vi "updateRobotExtraInfo.vi"(8 "error in (no error)":errorcluster, 9 "ReplayArray":bool[](array[boolean]), 11 "Game in":refnum<class "Game.lvclass">) -> (0 "error out":errorcluster, 1 "delay":dbl, 3 "Game out":refnum<class "Game.lvclass">)   [LabVIEW 2020, in "Game.lvclass"]
uses:
  Game.lvclass
  Robot_class/Robot.lvclass
  Game.lvclass/Game.ctl
  Team_class/Team.lvclass/Team.ctl
  Read AllyRef.vi
  Team_class/Read RobotRef.vi
  Read EnemyRef.vi
  Team_class/Write RobotRef.vi
  Write AllyRef.vi
  Write EnemyRef.vi
  Enemy_class/Enemy.lvclass
  Ally_class/Ally.lvclass
  Utilities_class/Utilities.lvclass
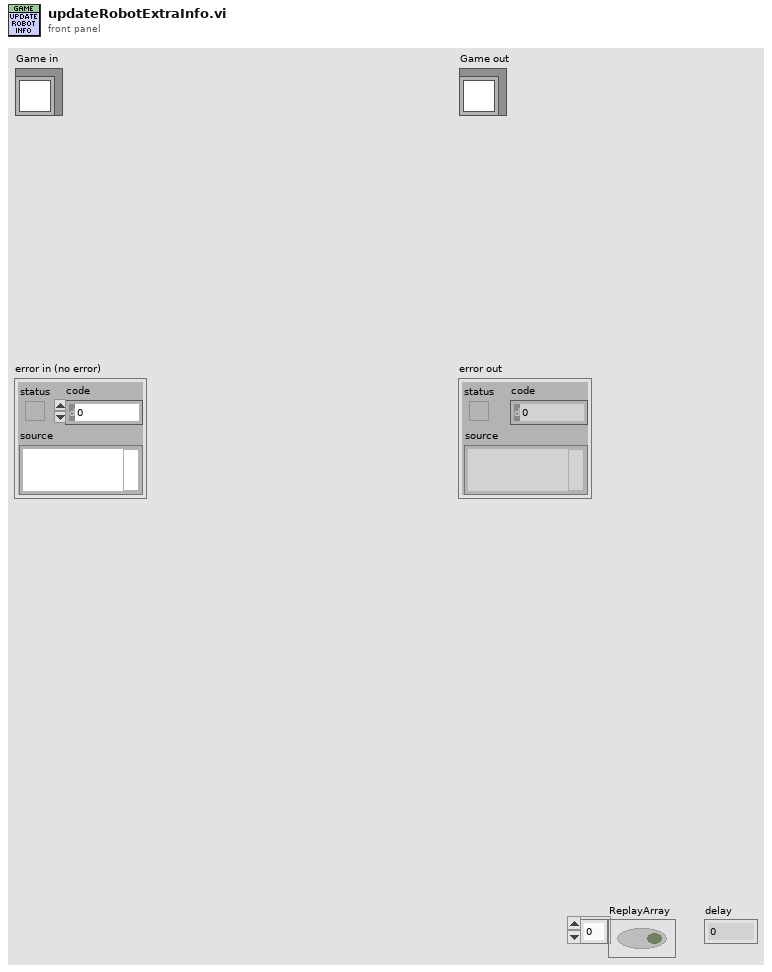
[diagram p1: front panel]
types:
  T1 = typedef "ReplayInfo.ctl" = cluster{"ByteArrayFromVision":u8[], "TimeStampSampledInReplay":string, "ByteArrayFromReferee":u8[], "AllyRobotExtraInfoArray":T2[], "EnemyRobotExtraInfoArray":T2[]}
  T2 = typedef "RobotExtraInfo.ctl" = cluster{"est_vx":dbl, "est_vy":dbl, "id":dbl}
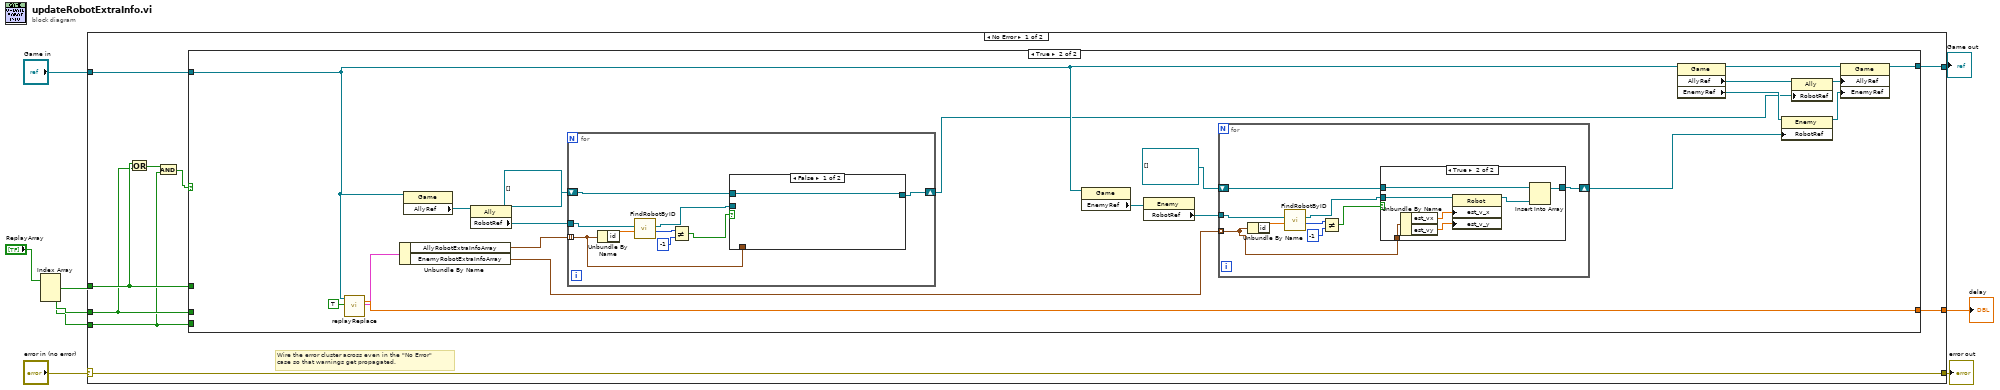
[diagram p0: block diagram]
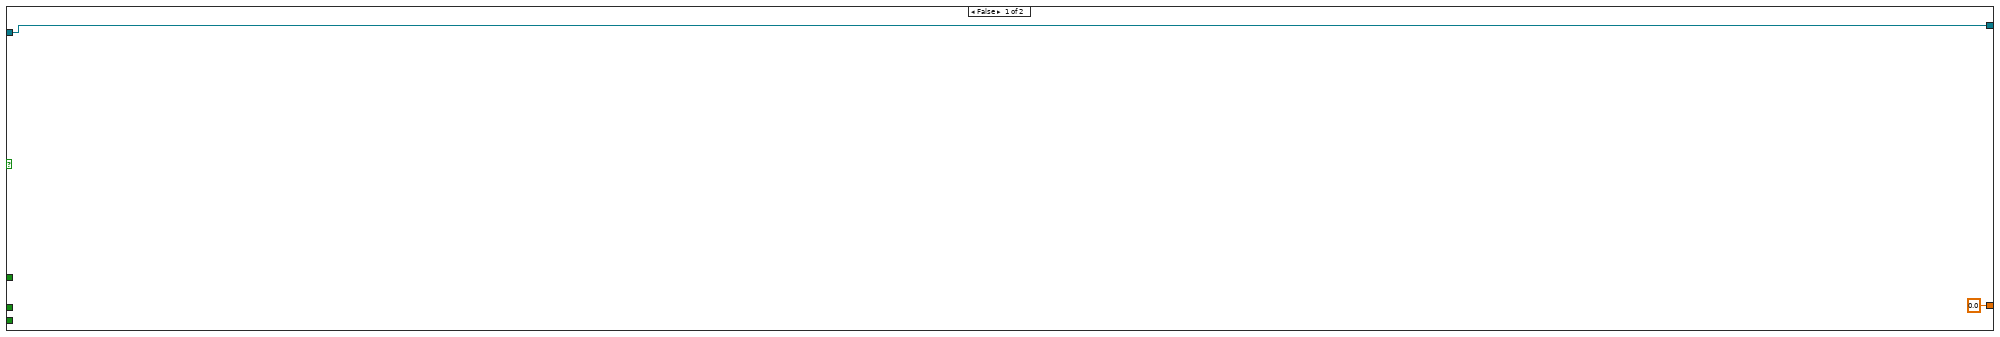
[diagram p2: hidden frame]
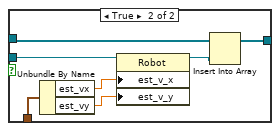
[diagram p4: hidden frame]
diagram:
  n1 = Index Array(array="ReplayArray") -> (element #1=w3:bool, element #2=w2:bool, element #3=w1:bool)  [unwired: 3 in]
  n2 = case shown="No Error" "error in (no error)" {
    selector: "error in (no error)" -> [w18 w76]
    tunnel: [w18 w76] -> w8
    tunnel: [w15 w75] -> w6
    tunnel: "Game in" -> [w16 w75]
    tunnel: w1 -> [w10 _]
    tunnel: w3 -> [w12 _]
    tunnel: w2 -> [w11 _]
    tunnel: [w17 _] -> w5
    frame No Error {
      # "Wire the error cluster across even in the \"No Error\"\ncase so that warnings get propagated."
      n3 = Or(x=w12, y=w11) -> (x .or. y?=w13:bool)
      n4 = And(x=w13, y=w10) -> (x .and. y?=w14:bool)
      n5 = case shown="True" w14 {
        tunnel: w10 -> [_ _]
        tunnel: w11 -> [_ _]
        tunnel: [0.0 ("delay") w39] -> w17
        tunnel: w12 -> [_ _]
        tunnel: w16 -> [w20 w29]
        tunnel: [w20 w21] -> w15
        frame False {
        }
        frame True {
          n6 = call "replayReplace.vi"("Game in"=w29, "vision?"=TRUE) -> ("delay"=w39:dbl, "ReplayInfo"=w34:T1)  [unwired: 12 in, 4 out]
          n7 = Unbundle By Name(w34) -> ("AllyRobotExtraInfoArray"=w33:T2[], "EnemyRobotExtraInfoArray"=w32:T2[])
          n8 = property class="Game"(reference=w29) -> ("AllyRef"=w38:refnum<class "Ally.lvclass">)  [unwired: 1 in, 2 out]
          n9 = property class="Ally"(reference=w38) -> ("RobotRef"=w37:refnum<class "Robot.lvclass">[])  [unwired: 1 in, 2 out]
          n10 = for {
            tunnel: w33 -> [w61] mode=indexing
            tunnel: w37 -> [w65]
            shift-right: [w58] -> w25
            shift-left: refnum<class "Robot.lvclass">[] [] ("RobotRef") -> [w59]
            n11 = Unbundle By Name(w61) -> ("id"=w66:dbl)
            n12 = call "FindRobotByID.vi"("id"=w66, "RobotRef"=w65) -> ("index"=w64:i32, "Robot"=w62:refnum<class "Robot.lvclass">)  [unwired: 6 in, 2 out]
            n13 = Not Equal?(x=w64, y=-1) -> (x != y?=w60:bool)
            n14 = case shown="False" w60 {
              tunnel: w62 -> [_ w73]
              tunnel: w61 -> [_ w74]
              tunnel: w59 -> [w67 w70]
              tunnel: [w67 w68] -> w58
              frame False {
              }
              frame True {
                n15 = Unbundle By Name(w74) -> ("est_vx"=w72:dbl, "est_vy"=w71:dbl)
                n16 = property class="Robot"(reference=w73, "est_v_x"=w72, "est_v_y"=w71) -> (reference out=w69:refnum<class "Robot.lvclass">)  [unwired: 1 in, 1 out]
                n17 = Insert Into Array(array=w70, new element=w69) -> (w68:refnum<class "Robot.lvclass">[])  [unwired: 1 in]
              }
            }
          }
          n18 = property class="Game"(reference=w29) -> ("EnemyRef"=w36:refnum<class "Enemy.lvclass">)  [unwired: 1 in, 2 out]
          n19 = property class="Enemy"(reference=w36) -> ("RobotRef"=w35:refnum<class "Robot.lvclass">[])  [unwired: 1 in, 2 out]
          n20 = for {
            tunnel: w35 -> [w48]
            tunnel: w32 -> [w43] mode=indexing
            shift-right: [w41] -> w26
            shift-left: refnum<class "Robot.lvclass">[] [] ("RobotRef") -> [w42]
            n21 = Unbundle By Name(w43) -> ("id"=w49:dbl)
            n22 = call "FindRobotByID.vi"("id"=w49, "RobotRef"=w48) -> ("index"=w47:i32, "Robot"=w46:refnum<class "Robot.lvclass">)  [unwired: 6 in, 2 out]
            n23 = Not Equal?(x=w47, y=-1) -> (x != y?=w44:bool)
            n24 = case shown="True" w44 {
              tunnel: w46 -> [_ w57]
              tunnel: w43 -> [_ w54]
              tunnel: w42 -> [w50 w53]
              tunnel: [w50 w51] -> w41
              frame False {
              }
              frame True {
                n25 = Unbundle By Name(w54) -> ("est_vx"=w56:dbl, "est_vy"=w55:dbl)
                n26 = property class="Robot"(reference=w57, "est_v_x"=w56, "est_v_y"=w55) -> (reference out=w52:refnum<class "Robot.lvclass">)  [unwired: 1 in, 1 out]
                n27 = Insert Into Array(array=w53, new element=w52) -> (w51:refnum<class "Robot.lvclass">[])  [unwired: 1 in]
              }
            }
          }
          n28 = property class="Game"(reference=w29) -> (reference out=w24:refnum<class "Game.lvclass">, "AllyRef"=w28:refnum<class "Ally.lvclass">, "EnemyRef"=w27:refnum<class "Enemy.lvclass">)  [unwired: 1 in, 1 out]
          n29 = property class="Enemy"(reference=w27, "RobotRef"=w26) -> (reference out=w22:refnum<class "Enemy.lvclass">)  [unwired: 1 in, 1 out]
          n30 = property class="Ally"(reference=w28, "RobotRef"=w25) -> (reference out=w23:refnum<class "Ally.lvclass">)  [unwired: 1 in, 1 out]
          n31 = property class="Game"(reference=w24, "AllyRef"=w23, "EnemyRef"=w22) -> (reference out=w21:refnum<class "Game.lvclass">)  [unwired: 1 in, 1 out]
        }
      }
    }
    frame Error {
    }
  }
  "error out" <- w8
  "Game out" <- w6
  "delay" <- w5
